vi "Check Scope on-board memory.vi"(0 "Scope":string, 5 "Acquisition Time":dbl, 11 "error in (no error)":errorcluster) -> (4 "IVI Refnum out":refnum<k15>, 6 "Required Record Length":i32, 8 "Maximum Record Length":i32=32000000, 10 "Insufficient Memory?":bool, 15 "error out":errorcluster)   [LabVIEW 2020, in "LDO Load Transient.lvlib"]
uses:
  LDO Load Transient.lvlib
  59f03915-b6bb-47a8-b10c-82860c18f887.vi
  <userlib>/_Soliton/Measurement Suite/Reusables/InstrumentSessionAPIs/SessionManagerApiPath.vi
  <vilib>/Utility/sysdir.llb/Get System Directory.vi
  <vilib>/Utility/LVLibp/Get Exported File Path.vi
  <userlib>/_Soliton/Measurement Suite/Reusables/Errors/Error 6001.vi
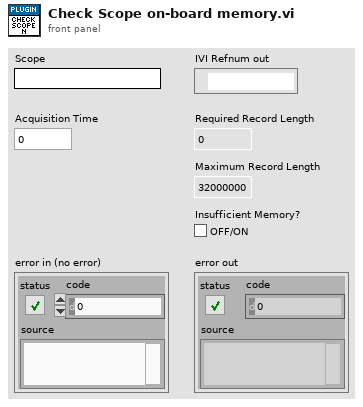
[diagram p1: front panel]
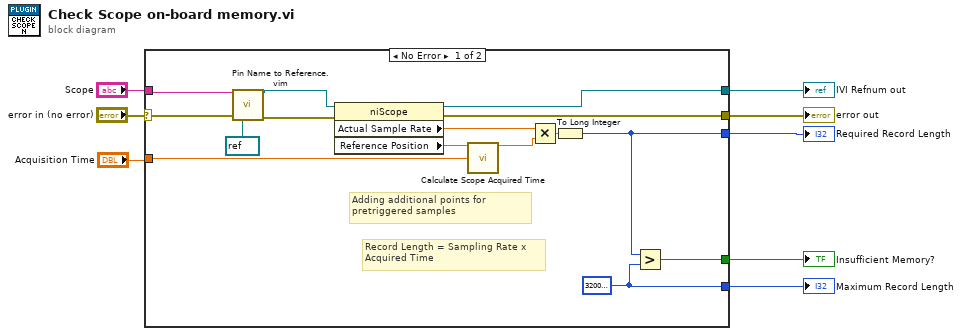
[diagram p0: block diagram]
diagram:
  n1 = case shown="No Error" "error in (no error)" {
    selector: "error in (no error)" -> [w12 w24]
    tunnel: "Acquisition Time" -> [w23 _]
    tunnel: [w18 w25] -> w7
    tunnel: "Scope" -> [w9 w25]
    tunnel: [w17 w24] -> w5
    tunnel: [w16 _] -> w3
    tunnel: [w15 _] -> w2
    tunnel: [w14 _] -> w1
    frame No Error {
      w15 = 32000000 ("y")
      # "Adding additional points for \npretriggered samples"
      # "Record Length = Sampling Rate x \nAcquired Time"
      n2 = call "Pin Name to Reference.vim"("Pin Name"=w9, "type"=refnum<k15> refnum ("instrument handle"), "error in (no error)"=w12) -> ("Reference"=w10:refnum<k15>, "error out"=w11:errorcluster)  [unwired: 7 in, 4 out]
      n3 = property class="niScope"(reference=w10, error in=w11) -> (reference out=w18:refnum<k15>, error out=w17:errorcluster, "Actual Sample Rate"=w21:dbl, "Reference Position"=w22:dbl)
      n4 = call "Calculate Scope Acquired Time.vi"("Scope Reference Position"=w22, "Acquisition Time"=w23) -> ("Scope Acquired Time"=w20:dbl)  [unwired: 13 in]
      n5 = Multiply(x=w21, y=w20) -> (x*y=w19:dbl)
      n6 = To Long Integer(number=w19) -> (32bit integer=w16:i32)
      n7 = Greater?(x=w16, y=w15) -> (0:w14:bool)
    }
    frame Error {
    }
  }
  "Required Record Length" <- w3
  "IVI Refnum out" <- w7
  "error out" <- w5
  "Maximum Record Length" <- w2
  "Insufficient Memory?" <- w1
